vi "rs3 init all.vi"(8 "error in":errorcluster, 10 "Select Device":i32, 11 "Select Sensor":i32) -> (0 "error out":errorcluster, 1 "Adv. enable?":i32, 2 "init results":T3, 3 "init error":string, 4 "All Devices":T2(array[cluster]), 5 "Sensor Array":T1(array[cluster]), 7 "Found RealSense":bool)   [LabVIEW 2018, in "libRealSense3.lvlib"]
doc: "Initialized the RealSense device. \nSelect the specific DEVICE and its specific SENSOR. \n\n\nINPUT:\nSelect Device The INDEX to the specific DEVICE handle\nSelect Sensor The INDEX to the specific SENSOR that is part of the selected DEVICE.\n \nOUTPUT:\ninit result Contains all the information about the selected device and its sensor. You will need to use the Dev Out HANDLE to communicate with the device. \n \nselected sensor array Contains the arrays of SENSORS attached to a specific DEVICE.\nall devices Contains array of all device that are attached to the PC."
uses:
  libRealSense3.lvlib
panel:
  # "RS3 Init All"
  # "(C) Intel Corp. 2017,  AGJ"
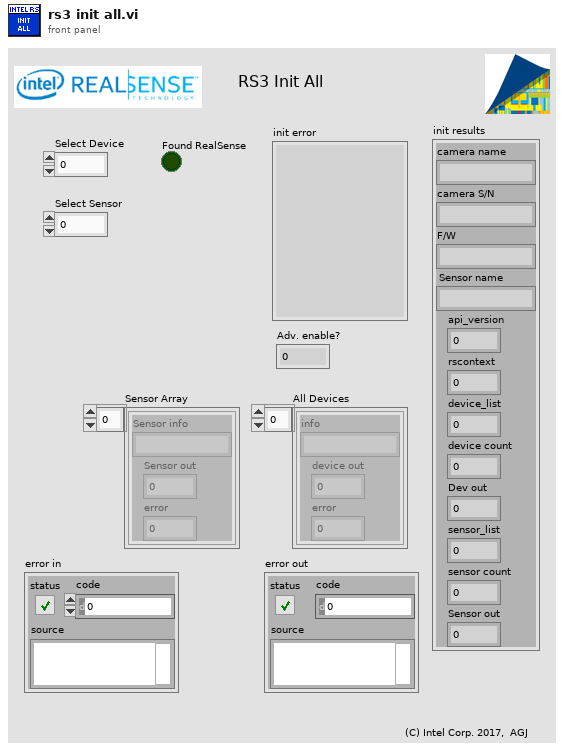
[diagram p1: front panel]
types:
  T1 = cluster{"Sensor info":string, "Sensor out":u64, "error":u64}[]
  T2 = cluster{"info":string, "device out":u64, "error":u64}[]
  T3 = cluster{"camera name":string, "camera S/N":string, "F/W":string, "Sensor name":string, "api_version":i32, "rscontext":u64, "device_list":u64, "device count":i32, "Dev out":u64, "sensor_list":u64, "sensor count":i32, "Sensor out":u64}
  T4 = cluster{"info":string, "device out":u64, "error":u64}
  T5 = cluster{"info":string, "info":string, "info":string, "Sensor info":string, "api_version":i32, "rscontext":u64, "device_list":u64, "device count":i32, "device out":u64, "sensor_list":u64, "sensor count":i32, "Sensor out":u64}
  T6 = cluster{"Sensor info":string, "Sensor out":u64, "error":u64}
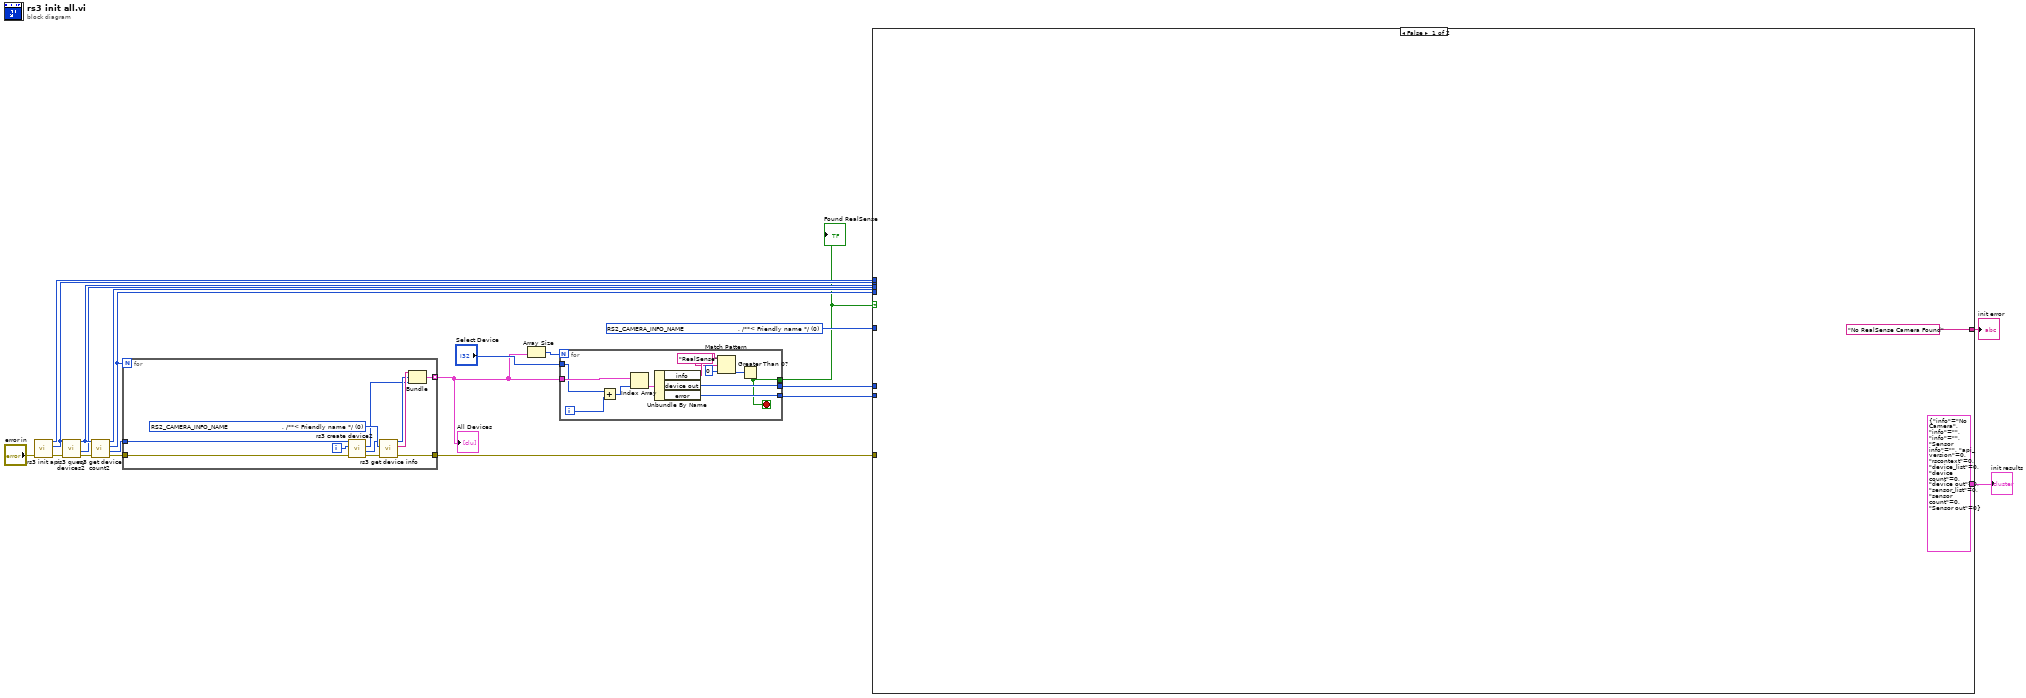
[diagram p0: block diagram]
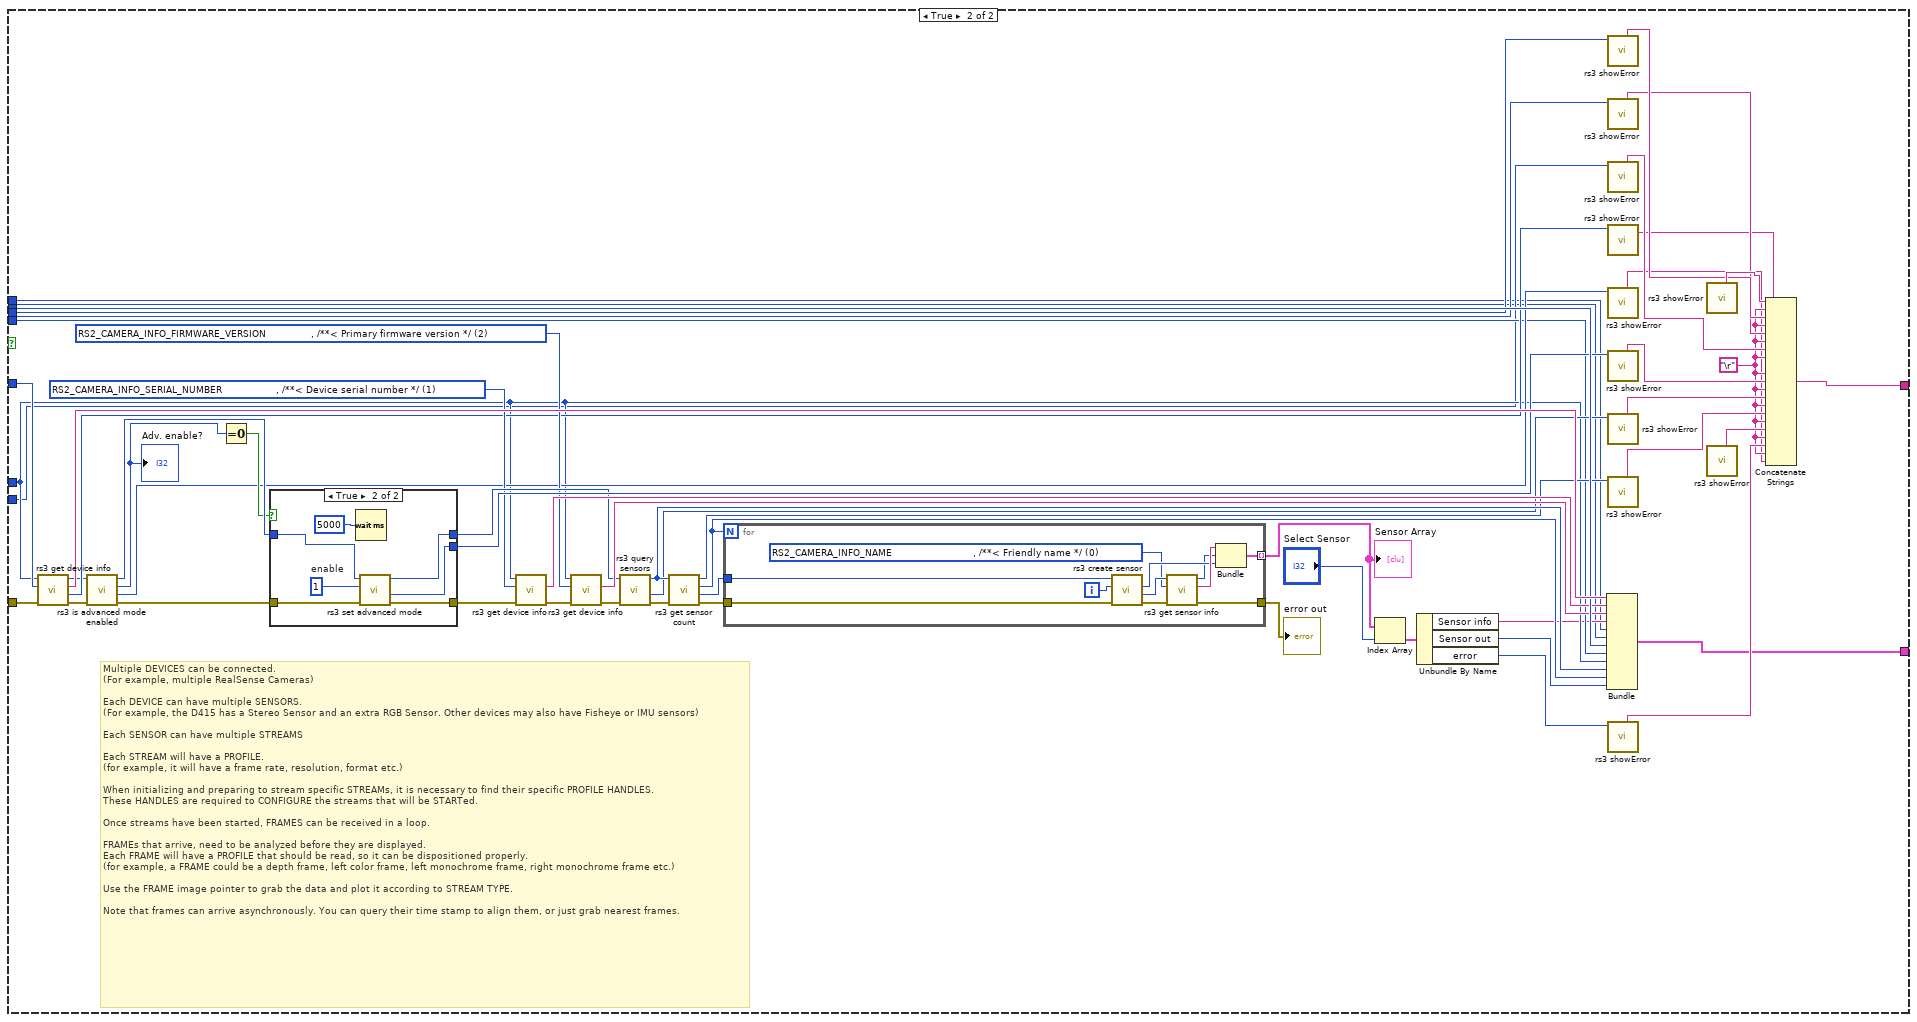
[diagram p2: hidden frame]
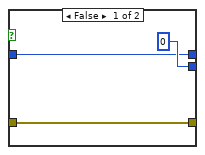
[diagram p3: hidden frame]
diagram:
  w20 = u16 0 items=["    RS2_CAMERA_INFO_NAME                           , /**< Friendly name */", "    RS2_CAMERA_INFO_SERIAL_NUMBER                  , /**< Device serial number */", "    RS2_CAMERA_INFO_FIRMWARE_VERSION               , /**< Primary firmware version */", "    RS2_CAMERA_INFO_PHYSICAL_PORT                       , /**< Unique identifier of the port the device is connected to (platform specific) */", "    RS2_CAMERA_INFO_DEBUG_OP_CODE                  , /**< If device supports firmware logging, this is the command to send to get logs from firmware */", "    RS2_CAMERA_INFO_ADVANCED_MODE                  , /**< True iff the device is in advanced mode */", "    RS2_CAMERA_INFO_PRODUCT_ID                     , /**< Product ID as reported in the USB descriptor */", "    RS2_CAMERA_INFO_CAMERA_LOCKED                  , /**< True iff EEPROM is locked */", "    RS2_CAMERA_INFO_COUNT                            /**< Number of enumeration values. Not a valid input: intended to be used in for-loops. */"] ("RS Camera info")
  n1 = call "rs3 init api.vi"("error in (no error)"="error in") -> ("error out"=w9:errorcluster, "rscontext"=w7:u64, "api_version"=w6:i32)  [unwired: 7 in, 1 out]
  n2 = call "rs3 query devices2.vi"("error in (no error)"=w9, "rscontext"=w7) -> ("error out"=w18:errorcluster, "error"=w17:u64, "device_list"=w21:u64)  [unwired: 7 in]
  n3 = call "rs3 get device count2.vi"("error in"=w18, "device_list"=w21) -> ("error out"=w12:errorcluster, "device_list_out"=w15:u64, "device count"=w16:i32, "error"=w19:u64)  [unwired: 6 in]
  n4 = for {
    N: w16 -> [_]
    tunnel: w15 -> [w32]
    tunnel: [w26] -> w1 mode=indexing
    tunnel: w12 -> [w25]
    tunnel: [w24] -> w11
    i -> [w31]
    w29 = u16 0 items=["    RS2_CAMERA_INFO_NAME                           , /**< Friendly name */", "    RS2_CAMERA_INFO_SERIAL_NUMBER                  , /**< Device serial number */", "    RS2_CAMERA_INFO_FIRMWARE_VERSION               , /**< Primary firmware version */", "    RS2_CAMERA_INFO_PHYSICAL_PORT                       , /**< Unique identifier of the port the device is connected to (platform specific) */", "    RS2_CAMERA_INFO_DEBUG_OP_CODE                  , /**< If device supports firmware logging, this is the command to send to get logs from firmware */", "    RS2_CAMERA_INFO_ADVANCED_MODE                  , /**< True iff the device is in advanced mode */", "    RS2_CAMERA_INFO_PRODUCT_ID                     , /**< Product ID as reported in the USB descriptor */", "    RS2_CAMERA_INFO_CAMERA_LOCKED                  , /**< True iff EEPROM is locked */", "    RS2_CAMERA_INFO_COUNT                            /**< Number of enumeration values. Not a valid input: intended to be used in for-loops. */"] ("RS Camera info")
    n5 = call "rs3 create device2.vi"("error in (no error)"=w25, "Device index"=w31, "device list in"=w32) -> ("error out"=w30:errorcluster, "Dev out"=w23:u64, "error"=w22:u64)  [unwired: 5 in, 1 out]
    n6 = call "rs3 get device info.vi"("error in (no error)"=w30, "RS Camera info"=w29, "device in"=w23) -> ("error out"=w24:errorcluster, "info"=w28:string, "device out"=w27:u64)  [unwired: 5 in, 1 out]
    n7 = Bundle("info"=w28, "device out"=w27, "error"=w22) -> (w26:T4)  [unwired: 1 in]
  }
  "All Devices" <- w1
  n8 = Array Size(array=w1) -> (size(s)=w2:i32)
  n9 = for {
    N: w2 -> [_]
    tunnel: w1 -> [w44]
    tunnel: "Select Device" -> [w35]
    tunnel: [w42] -> w13
    tunnel: [w41] -> w10
    tunnel: [w33] -> w5
    i -> [w36]
    stop <- w33 stop-if-true
    n10 = Add(x=w35, y=w36) -> (x+y=w37:i32)
    n11 = Index Array(array=w44, index=w37) -> (element=w43:T4)
    n12 = Unbundle By Name(w43) -> ("info"=w39:string, "device out"=w42:u64, "error"=w41:u64)
    n13 = Match Pattern(string=w39, regular expression="RealSense" ("string"), offset (0)=0) -> (offset past match=w34:i32)  [unwired: 3 out]
    n14 = Greater Than 0?(x=w34) -> (x > 0?=w33:bool)
  }
  "Found RealSense" <- w5
  n15 = case shown="False" w5 {
    tunnel: w21 -> [_ w100]
    tunnel: w20 -> [_ w87]
    tunnel: w19 -> [_ w85]
    tunnel: w17 -> [_ w84]
    tunnel: w16 -> [_ w64]
    tunnel: w13 -> [_ w63]
    tunnel: w11 -> [_ w62]
    tunnel: w10 -> [_ w61]
    tunnel: w7 -> [_ w50]
    tunnel: w6 -> [_ w49]
    tunnel: ["No RealSense Camera Found" w48] -> w4
    tunnel: [T5 {"info"="No Camera", "info"="", "info"="", "Sensor info"="", "api_version"=0, "rscontext"=0, "device_list"=0, "device count"=0, "device out"=0, "sensor_list"=0, "sensor count"=0, "Sensor out"=0} w47] -> w3
    frame False {
    }
    frame True {
      w66 = "\r"
      w94 = u16 2 items=["    RS2_CAMERA_INFO_NAME                           , /**< Friendly name */", "    RS2_CAMERA_INFO_SERIAL_NUMBER                  , /**< Device serial number */", "    RS2_CAMERA_INFO_FIRMWARE_VERSION               , /**< Primary firmware version */", "    RS2_CAMERA_INFO_PHYSICAL_PORT                       , /**< Unique identifier of the port the device is connected to (platform specific) */", "    RS2_CAMERA_INFO_DEBUG_OP_CODE                  , /**< If device supports firmware logging, this is the command to send to get logs from firmware */", "    RS2_CAMERA_INFO_ADVANCED_MODE                  , /**< True iff the device is in advanced mode */", "    RS2_CAMERA_INFO_PRODUCT_ID                     , /**< Product ID as reported in the USB descriptor */", "    RS2_CAMERA_INFO_CAMERA_LOCKED                  , /**< True iff EEPROM is locked */", "    RS2_CAMERA_INFO_COUNT                            /**< Number of enumeration values. Not a valid input: intended to be used in for-loops. */"] ("RS Camera info")
      w93 = u16 1 items=["    RS2_CAMERA_INFO_NAME                           , /**< Friendly name */", "    RS2_CAMERA_INFO_SERIAL_NUMBER                  , /**< Device serial number */", "    RS2_CAMERA_INFO_FIRMWARE_VERSION               , /**< Primary firmware version */", "    RS2_CAMERA_INFO_PHYSICAL_PORT                       , /**< Unique identifier of the port the device is connected to (platform specific) */", "    RS2_CAMERA_INFO_DEBUG_OP_CODE                  , /**< If device supports firmware logging, this is the command to send to get logs from firmware */", "    RS2_CAMERA_INFO_ADVANCED_MODE                  , /**< True iff the device is in advanced mode */", "    RS2_CAMERA_INFO_PRODUCT_ID                     , /**< Product ID as reported in the USB descriptor */", "    RS2_CAMERA_INFO_CAMERA_LOCKED                  , /**< True iff EEPROM is locked */", "    RS2_CAMERA_INFO_COUNT                            /**< Number of enumeration values. Not a valid input: intended to be used in for-loops. */"] ("RS Camera info")
      # "Multiple DEVICES can be connected. \n(For example, multiple RealSense Cameras)\n\nEach DEVICE can have multiple SENSORS. \n(For example, the D415 has a Stereo Sensor and an extra RGB Sensor. Other devices may also have Fisheye or IMU sensors) \n\nEach SENSOR can have multiple STREAMS\n\nEach STREAM will have a PROFILE. \n(for example, it will have a frame rate, resolution, format etc.)\n\nWhen initializing and preparing to stream specific STREAMs, it is necessary to find their specific PROFILE HANDLES.\nThese HANDLES are required to CONFIGURE the streams that will be STARTed. \n\nOnce streams have been started, FRAMES can be received in a loop. \n \nFRAMEs that arrive, need to be analyzed before they are displayed. \nEach FRAME will have a PROFILE that should be read, so it can be dispositioned properly.\n(for example, a FRAME could be a depth frame, left color frame, left monochrome frame, right monochrome frame etc.)\n\nUse the FRAME image pointer to grab the data and plot it according to STREAM TYPE.\n\nNote that frames can arrive asynchronously. You can query their time stamp to align them, or just grab nearest frames."
      n16 = call "rs3 get device info.vi"("error in (no error)"=w62, "RS Camera info"=w87, "device in"=w63) -> ("error out"=w73:errorcluster, "error"=w86:u64, "info"=w101:string, "device out"=w71:u64)  [unwired: 5 in]
      n17 = call "rs3 is advanced mode enabled.vi"("error in (no error)"=w73, "device in"=w71) -> ("error out"=w72:errorcluster, "error"=w67:u64, "enable?"=w69:i32, "device out"=w70:u64)  [unwired: 6 in]
      "Adv. enable?" <- w69
      n18 = Equal To 0?(x=w69) -> (x = 0?=w68:bool)
      n19 = case shown="True" w68 {
        tunnel: [u64 0 ("error") w123] -> w97
        tunnel: [w114 w121] -> w96
        tunnel: w70 -> [w114 w120]
        tunnel: [w116 w119] -> w95
        tunnel: w72 -> [w116 w118]
        frame False {
        }
        frame True {
          w122 = 1  # enable
          n20 = Wait (ms)(milliseconds to wait=u32 5000) -> ()  [unwired: 1 out]
          n21 = call "rs3 set advanced mode.vi"("error in (no error)"=w118, "enable"=w122, "device in"=w120) -> ("error out"=w119:errorcluster, "error"=w123:u64, "device out"=w121:u64)  [unwired: 6 in]
        }
      }
      n22 = call "rs3 get device info.vi"("error in (no error)"=w95, "RS Camera info"=w93, "device in"=w63) -> ("error out"=w91:errorcluster, "info"=w98:string)  [unwired: 5 in, 2 out]
      n23 = call "rs3 get device info.vi"("error in (no error)"=w91, "RS Camera info"=w94, "device in"=w63) -> ("error out"=w92:errorcluster, "info"=w99:string)  [unwired: 5 in, 2 out]
      n24 = call "rs3 query sensors.vi"("error in (no error)"=w92, "device in"=w96) -> ("error out"=w89:errorcluster, "error"=w88:u64, "sensor_list"=w102:u64)  [unwired: 7 in]
      n25 = call "rs3 get sensor count.vi"("error in"=w89, "sensor_list"=w102) -> ("error out"=w59:errorcluster, "sensor_list_out"=w58:u64, "sensor count"=w60:i32, "error"=w90:u64)  [unwired: 6 in]
      n26 = for {
        N: w60 -> [_]
        tunnel: w59 -> [w113]
        tunnel: w58 -> [w110]
        tunnel: [w104] -> w57 mode=indexing
        tunnel: [w103] -> w52
        i -> [w111]
        w106 = u16 0 items=["    RS2_CAMERA_INFO_NAME                           , /**< Friendly name */", "    RS2_CAMERA_INFO_SERIAL_NUMBER                  , /**< Device serial number */", "    RS2_CAMERA_INFO_FIRMWARE_VERSION               , /**< Primary firmware version */", "    RS2_CAMERA_INFO_PHYSICAL_PORT                       , /**< Unique identifier of the port the device is connected to (platform specific) */", "    RS2_CAMERA_INFO_DEBUG_OP_CODE                  , /**< If device supports firmware logging, this is the command to send to get logs from firmware */", "    RS2_CAMERA_INFO_ADVANCED_MODE                  , /**< True iff the device is in advanced mode */", "    RS2_CAMERA_INFO_PRODUCT_ID                     , /**< Product ID as reported in the USB descriptor */", "    RS2_CAMERA_INFO_CAMERA_LOCKED                  , /**< True iff EEPROM is locked */", "    RS2_CAMERA_INFO_COUNT                            /**< Number of enumeration values. Not a valid input: intended to be used in for-loops. */"] ("RS Sensor info")
        n27 = call "rs3 create sensor.vi"("error in (no error)"=w113, "Sensor index"=w111, "Sensor list"=w110) -> ("error out"=w112:errorcluster, "Sensor out"=w108:u64, "error"=w107:u64)  [unwired: 5 in, 1 out]
        n28 = call "rs3 get sensor info.vi"("error in (no error)"=w112, "RS Camera info"=w106, "Sensor in"=w108) -> ("error out"=w103:errorcluster, "Sensor info"=w109:string, "Sensor out"=w105:u64)  [unwired: 5 in, 1 out]
        n29 = Bundle("Sensor info"=w109, "Sensor out"=w105, "error"=w107) -> (w104:T6)  [unwired: 1 in]
      }
      "error out" <- w52
      "Sensor Array" <- w57
      n30 = Index Array(array=w57, index="Select Sensor") -> (element=w55:T6)
      n31 = Unbundle By Name(w55) -> ("Sensor info"=w51:string, "Sensor out"=w54:u64, "error"=w53:u64)
      n32 = Bundle("info"=w101, "info"=w98, "info"=w99, "Sensor info"=w51, "api_version"=w49, "rscontext"=w50, "device_list"=w100, "device count"=w64, "device out"=w63, "sensor_list"=w102, "sensor count"=w60, "Sensor out"=w54) -> (w47:T5)  [unwired: 1 in]
      n33 = call "rs3 showError.vi"("error"=w84) -> ("Error summary"=w82:string)  [unwired: 6 in, 4 out]
      n34 = call "rs3 showError.vi"("error"=w85) -> ("Error summary"=w81:string)  [unwired: 6 in, 4 out]
      n35 = call "rs3 showError.vi"("error"=w61) -> ("Error summary"=w80:string)  [unwired: 6 in, 4 out]
      n36 = call "rs3 showError.vi"("error"=w86) -> ("Error summary"=w79:string)  [unwired: 6 in, 4 out]
      n37 = call "rs3 showError.vi"("error"=w67) -> ("Error summary"=w65:string)  [unwired: 6 in, 4 out]
      n38 = call "rs3 showError.vi"("error"=w97) -> ("Error summary"=w78:string)  [unwired: 6 in, 4 out]
      n39 = call "rs3 showError.vi"("error"=w88) -> ("Error summary"=w77:string)  [unwired: 6 in, 4 out]
      n40 = call "rs3 showError.vi"("error"=w90) -> ("Error summary"=w76:string)  [unwired: 6 in, 4 out]
      n41 = call "rs3 showError.vi"("error"=w53) -> ("Error summary"=w74:string)  [unwired: 6 in, 4 out]
      n42 = call "rs3 showError.vi"() -> ("Error summary"=w83:string)  [unwired: 7 in, 4 out]
      n43 = call "rs3 showError.vi"() -> ("Error summary"=w75:string)  [unwired: 7 in, 4 out]
      n44 = Concatenate Strings(w83, w66, w82, w66, w81, w66, w80, w66, w79, w66, w78, w66, w77, w66, w76, w66, w75, w66, w74, w66, w65) -> (w48:string)
    }
  }
  "init error" <- w4
  "init results" <- w3
